vi "S2C_OM8257_Poly_RUN.vi"(8 "Error In":errorcluster, 10 "RUN":T1={"Voltage-Hi (V)"=125.0, "Voltage-Lo (V)"=0.0, "Amp-Hi (A)"=10.0, "Amp-Lo (A)"=0.0, "Dwell (s)"=1.0, "Delay (s)"=0.2, "Leakage-Hi (mA)"=10.0, "Leakage-Lo (mA)"=0.0, "Power-Hi (W)"=1000, "Power-Lo (W)"=0, "PF-Hi"=1.0, "PF-Lo"=0.0, "AC Src Voltage (V)"=115.0, "AC Src A-Hi (A)"=0.0, "AC Source"=FALSE, "AC Src Frequency (Hz)"=60, "AC Src OC Fold"=FALSE, "AC Src Output"=TRUE, "AC Src Range"=TRUE, "Active Link"=FALSE, "Step Selection"=1, "Add Step"=FALSE, "P1P4C1Exe"=FALSE}, 11 "Settings":T2={"Driver"="Omnia8257", "Command"="CfgStep RUN", "Return"="ErrorStatus", "Parameters"="", "Timeout"=10.0}) -> (0 "Error Out":errorcluster, 3 "Response":string)   [LabVIEW 2015]
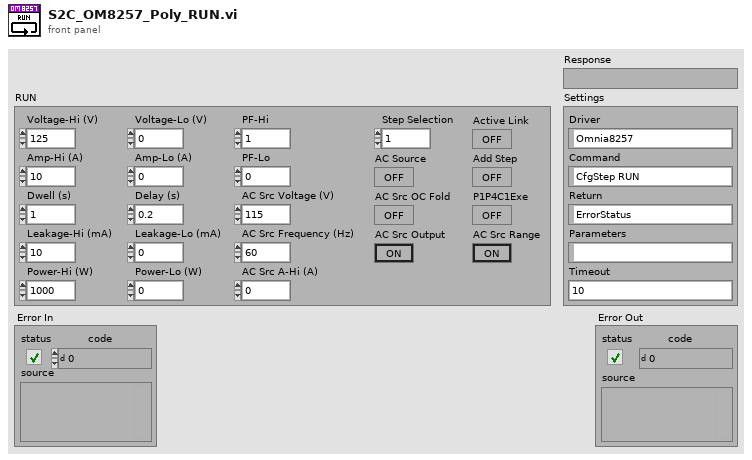
[diagram p1: front panel]
types:
  T1 = cluster{"Voltage-Hi (V)":dbl, "Voltage-Lo (V)":dbl, "Amp-Hi (A)":dbl, "Amp-Lo (A)":dbl, "Dwell (s)":dbl, "Delay (s)":dbl, "Leakage-Hi (mA)":dbl, "Leakage-Lo (mA)":dbl, "Power-Hi (W)":u16, "Power-Lo (W)":u16, "PF-Hi":dbl, "PF-Lo":dbl, "AC Src Voltage (V)":dbl, "AC Src A-Hi (A)":dbl, "AC Source":bool, "AC Src Frequency (Hz)":u16, "AC Src OC Fold":bool, "AC Src Output":bool, "AC Src Range":bool, "Active Link":bool, "Step Selection":i32, "Add Step":bool, "P1P4C1Exe":bool}
  T2 = cluster{"Driver":string, "Command":string, "Return":string, "Parameters":string, "Timeout":dbl}
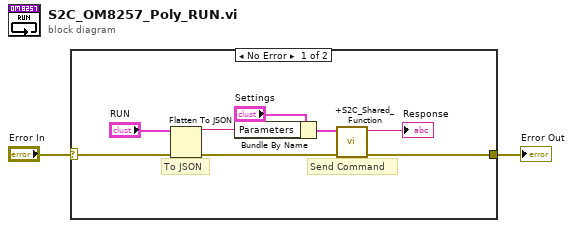
[diagram p0: block diagram]
diagram:
  n1 = case shown="No Error" "Error In" {
    selector: "Error In" -> [w6 w11]
    tunnel: [w5 w11] -> w1
    frame No Error {
      # "To JSON"
      # "Send Command"
      n2 = Flatten To JSON(anything="RUN", error in (no error)=w6) -> (JSON string=w7:string, 11:w9:errorcluster)  [unwired: 1 in]
      n3 = Bundle By Name(cluster="Settings", "Parameters"=w7) -> (w10:T2)
      n4 = call "+S2C_Shared_Function.vi"("Error In"=w9, "Settings"=w10) -> ("Error Out"=w5:errorcluster, "Response"=→"Response":string)  [unwired: 8 in]
    }
    frame Error {
    }
  }
  "Error Out" <- w1
